vi "operationFunction.vi"(1 "y":dbl, 2 "Operation":string(combo), 3 "x":dbl) -> (0 "Answer":dbl)   [LabVIEW 2018]
panel:
  out "Units":string
  in  "stop":bool
  out "Error Message":string
  in  "Radians/Degrees":bool
  out "Operation Taken":string
  # "Tom's Calculator"
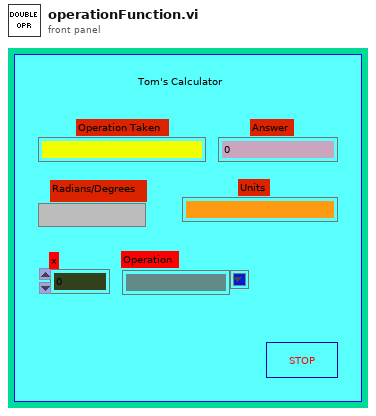
[diagram p1: front panel]
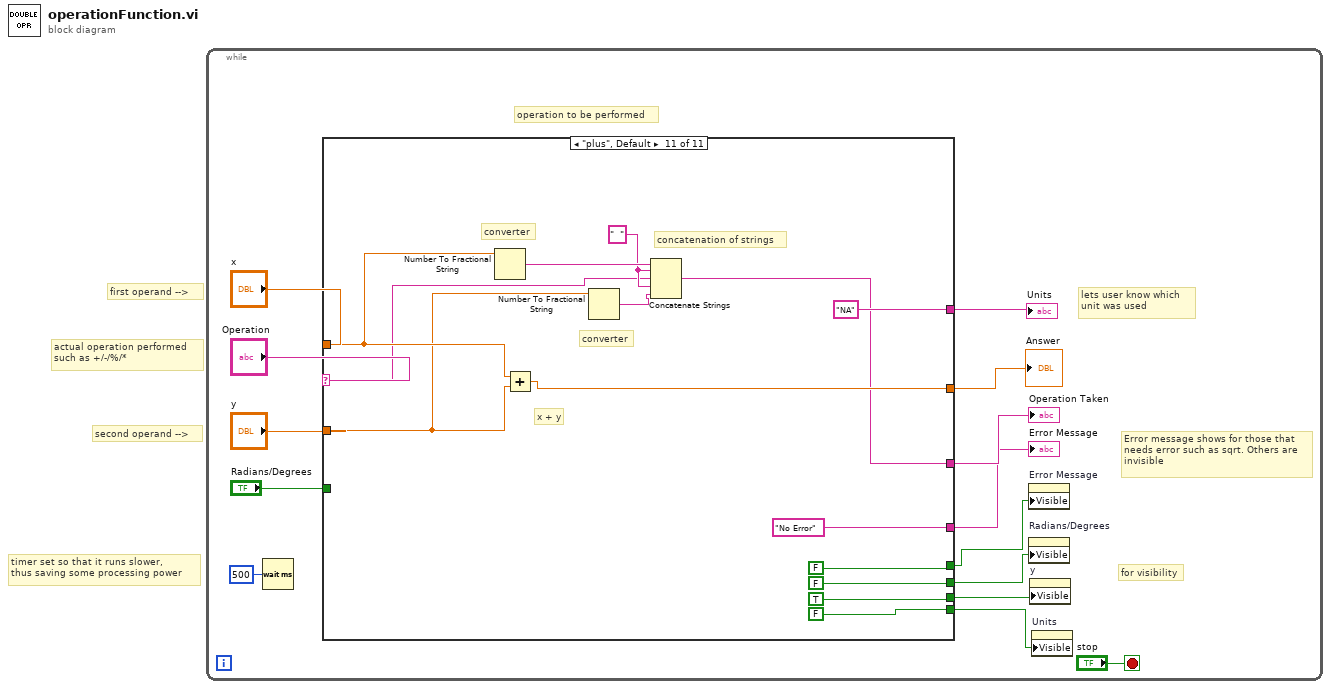
[diagram p0: block diagram]
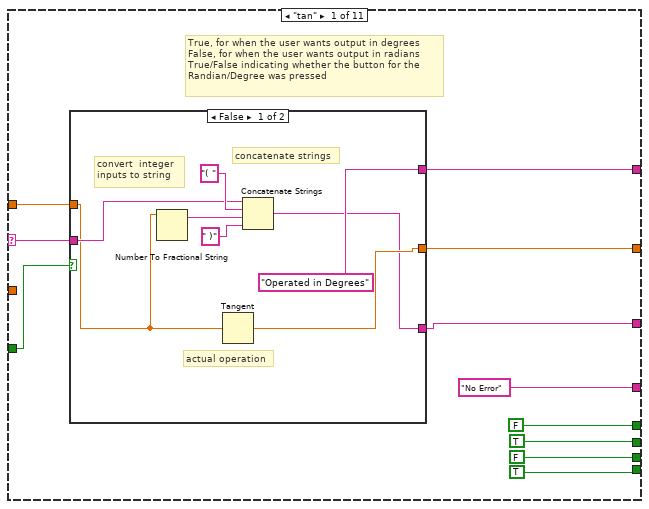
[diagram p2: hidden frame]
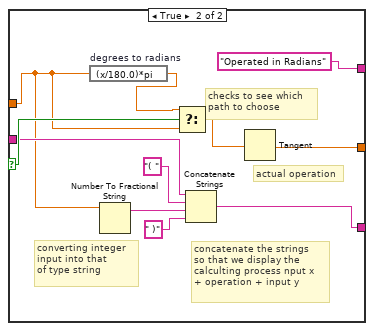
[diagram p3: hidden frame]
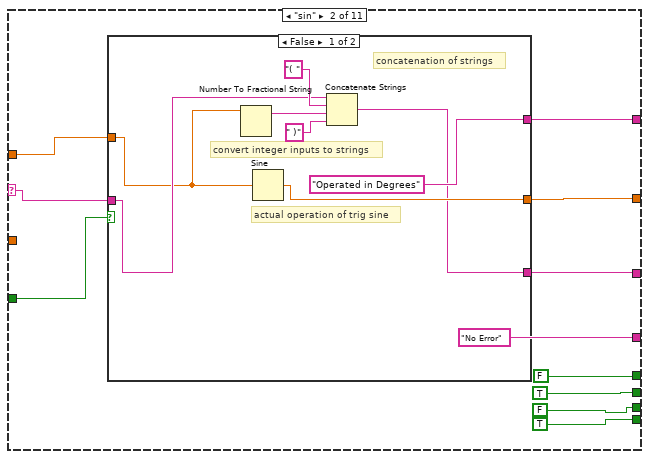
[diagram p4: hidden frame]
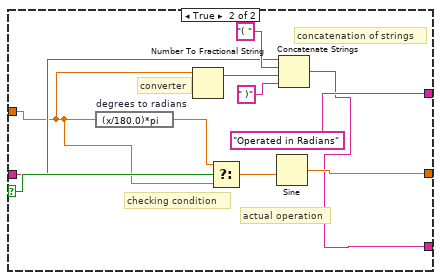
[diagram p5: hidden frame]
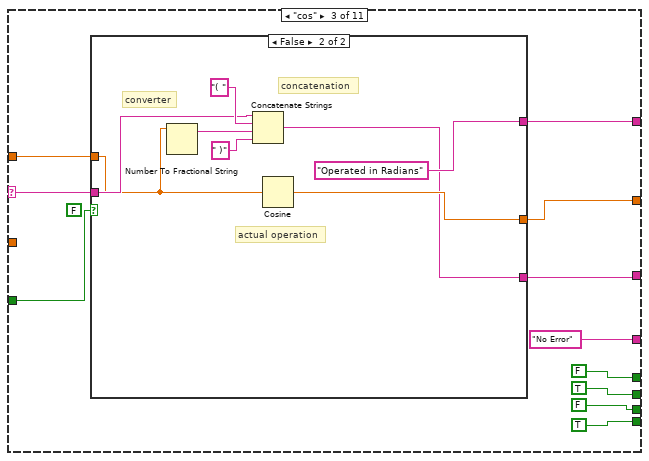
[diagram p6: hidden frame]
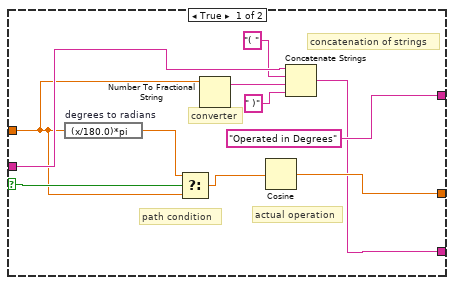
[diagram p7: hidden frame]
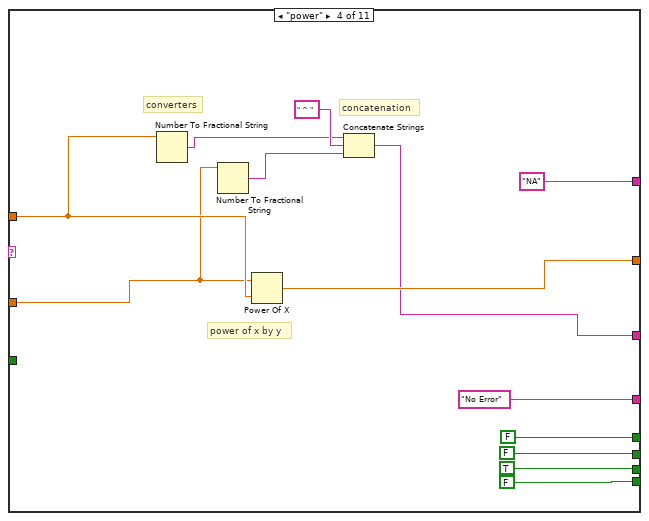
[diagram p8: hidden frame]
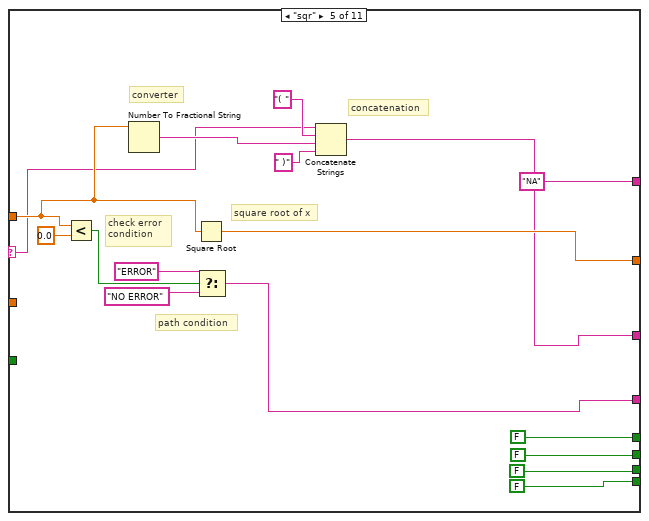
[diagram p9: hidden frame]
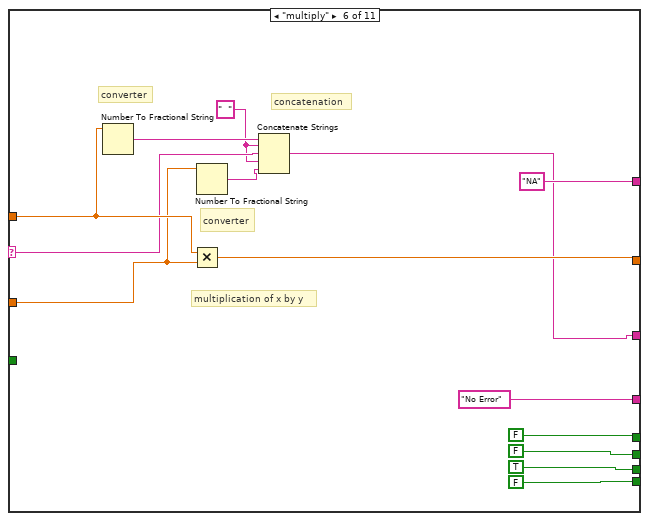
[diagram p10: hidden frame]
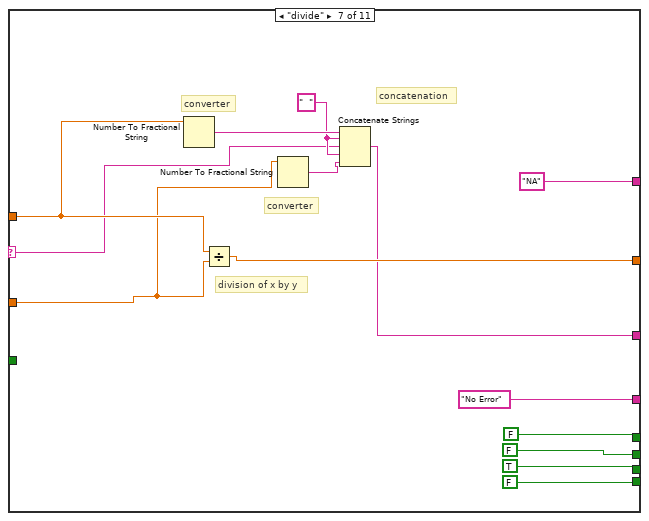
[diagram p11: hidden frame]
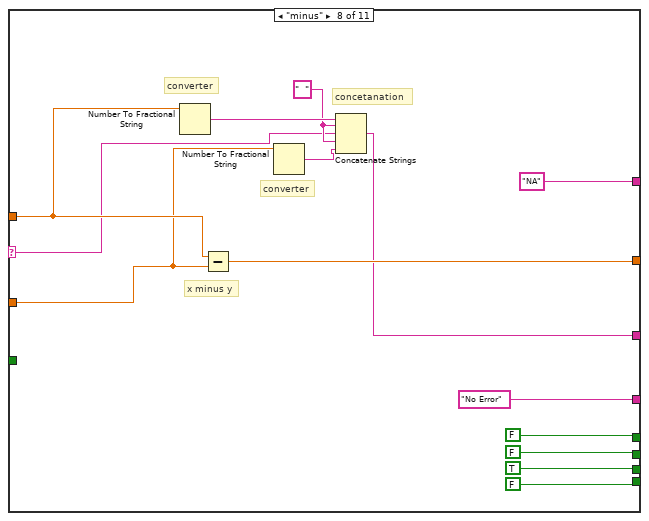
[diagram p12: hidden frame]
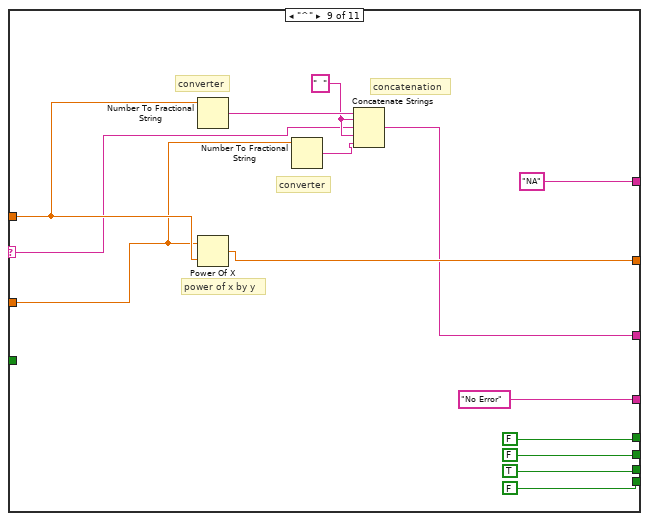
[diagram p13: hidden frame]
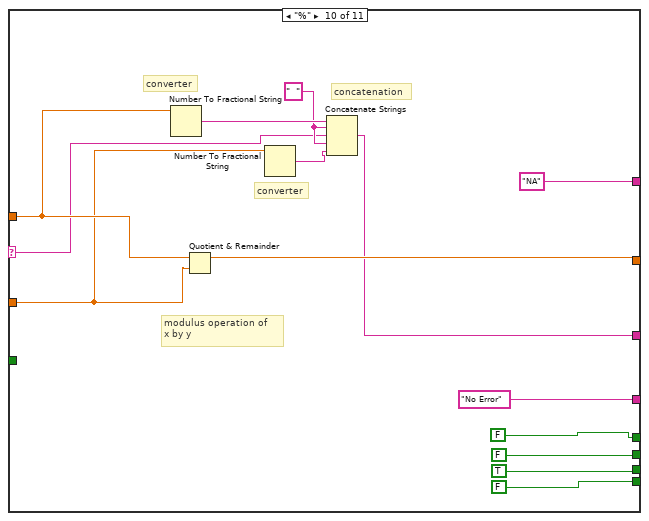
[diagram p14: hidden frame]
diagram:
  # "timer set so that it runs slower,\nthus saving some processing power"
  # "actual operation performed \nsuch as +/-/%/*"
  # "second operand -->"
  # "first operand -->"
  n1 = while {
    stop <- "stop" stop-if-true
    # "for visibility"
    # "Error message shows for those that \nneeds error such as sqrt. Others are \ninvisible"
    # "lets user know which \nunit was used"
    # "operation to be performed"
    n2 = Wait (ms)(milliseconds to wait=u32 500) -> ()  [unwired: 1 out]
    n3 = case shown="\"plus\", Default" "Operation" {
      selector: "Operation" -> [w16 w52 w76 _ w118 w137 w151 w165 w178 w193 w205]
      tunnel: "x" -> [w25 w54 w85 w109 w122 w141 w152 w166 w180 w194 w208]
      tunnel: "y" -> [_ _ _ w107 _ w139 w150 w164 w179 w192 w207]
      tunnel: [w24 w55 w84 w117 w132 w148 w162 w176 w190 w204 w218] -> w10
      tunnel: [w15 w50 w75 w105 w119 w138 w149 w163 w177 w191 w206] -> w11
      tunnel: ["No Error" "No Error" "No Error" "No Error" w129 "No Error" "No Error" "No Error" "No Error" "No Error" "No Error"] -> w9
      tunnel: "Radians/Degrees" -> [w22 w51 w82 _ _ _ _ _ _ _ _]
      tunnel: [w21 w49 w81 "NA" "NA" "NA" "NA" "NA" "NA" "NA" "NA"] -> w5
      tunnel: [FALSE FALSE FALSE TRUE FALSE TRUE TRUE TRUE TRUE TRUE TRUE] -> w4
      tunnel: [TRUE TRUE TRUE FALSE FALSE FALSE FALSE FALSE FALSE FALSE FALSE] -> w3
      tunnel: [TRUE TRUE TRUE FALSE FALSE FALSE FALSE FALSE FALSE FALSE FALSE] -> w2
      tunnel: [FALSE FALSE FALSE FALSE FALSE FALSE FALSE FALSE FALSE FALSE FALSE] -> w1
      frame "tan" {
        # "True, for when the user wants output in degrees\nFalse, for when the user wants output in radians\nTrue/False indicating whether the button for the\nRandian/Degree was pressed"
        n4 = case shown="False" w22 {
          selector: w22 -> [_ w43]
          tunnel: w25 -> [w26 w34]
          tunnel: [w33 w44] -> w24
          tunnel: ["Operated in Degrees" "Operated in Radians"] -> w21
          tunnel: w16 -> [w28 w36]
          tunnel: [w27 w35] -> w15
          frame False {
            # "actual operation"
            # "convert  integer \ninputs to string"
            # "concatenate strings"
            n5 = Number To Fractional String(number=w26) -> (F-format string=w31:string)  [unwired: 3 in]
            n6 = Tangent(1:w26) -> (0:w33:dbl)
            n7 = Concatenate Strings(w28, "( " ("string"), w31, " )" ("string")) -> (w27:string)
          }
          frame True {
            # "converting integer \ninput into that \nof type string"
            # "actual operation"
            # "checks to see which \npath to choose"
            # "concatenate the strings\nso that we display the \ncalculting process nput x \n+ operation + input y"
            n8 = expression code="(x/180.0)*pi" "degrees to radians"(w34) -> (w42:dbl)
            n9 = Number To Fractional String(number=w34) -> (F-format string=w39:string)  [unwired: 3 in]
            n10 = Select(t=w42, s=w43, f=w34) -> (s? t:f=w41:dbl)
            n11 = Concatenate Strings(w36, "( " ("string"), w39, " )" ("string")) -> (w35:string)
            n12 = Tangent(1:w41) -> (0:w44:dbl)
          }
        }
      }
      frame "sin" {
        n13 = case shown="False" w51 {
          selector: w51 -> [_ w71]
          tunnel: [w63 w74] -> w55
          tunnel: w54 -> [w56 w65]
          tunnel: w52 -> [w58 w66]
          tunnel: [w57 w64] -> w50
          tunnel: ["Operated in Degrees" "Operated in Radians"] -> w49
          frame False {
            # "actual operation of trig sine"
            # "convert integer inputs to strings"
            # "concatenation of strings"
            n14 = Number To Fractional String(number=w56) -> (F-format string=w61:string)  [unwired: 3 in]
            n15 = Sine(x=w56) -> (sin(x)=w63:dbl)
            n16 = Concatenate Strings(w58, "( " ("string"), w61, " )" ("string")) -> (w57:string)
          }
          frame True {
            # "concatenation of strings"
            # "converter"
            # "checking condition"
            # "actual operation"
            n17 = expression code="(x/180.0)*pi" "degrees to radians"(w65) -> (w73:dbl)
            n18 = Number To Fractional String(number=w65) -> (F-format string=w69:string)  [unwired: 3 in]
            n19 = Select(t=w73, s=w71, f=w65) -> (s? t:f=w72:dbl)
            n20 = Sine(x=w72) -> (sin(x)=w74:dbl)
            n21 = Concatenate Strings(w66, "( " ("string"), w69, " )" ("string")) -> (w64:string)
          }
        }
      }
      frame "cos" {
        (unwired) FALSE
        n22 = case shown="False" w82 {
          selector: w82 -> [w96 _]
          tunnel: w85 -> [w86 w98]
          tunnel: [w94 w104] -> w84
          tunnel: ["Operated in Degrees" "Operated in Radians"] -> w81
          tunnel: [w87 w97] -> w75
          tunnel: w76 -> [w90 w99]
          frame True {
            # "concatenation of strings"
            # "converter"
            # "actual operation"
            # "path condition"
            n23 = expression code="(x/180.0)*pi" "degrees to radians"(w86) -> (w95:dbl)
            n24 = Select(t=w95, s=w96, f=w86) -> (s? t:f=w88:dbl)
            n25 = Number To Fractional String(number=w86) -> (F-format string=w92:string)  [unwired: 3 in]
            n26 = Cosine(x=w88) -> (cos(x)=w94:dbl)
            n27 = Concatenate Strings(w90, "( " ("string"), w92, " )" ("string")) -> (w87:string)
          }
          frame False {
            # "concatenation"
            # "converter"
            # "actual operation"
            n28 = Number To Fractional String(number=w98) -> (F-format string=w102:string)  [unwired: 3 in]
            n29 = Concatenate Strings(w99, "( " ("string"), w102, " )" ("string")) -> (w97:string)
            n30 = Cosine(x=w98) -> (cos(x)=w104:dbl)
          }
        }
      }
      frame "power" {
        # "concatenation"
        # "converters"
        # "power of x by y"
        n31 = Number To Fractional String(number=w109) -> (F-format string=w108:string)  [unwired: 3 in]
        n32 = Number To Fractional String(number=w107) -> (F-format string=w106:string)  [unwired: 3 in]
        n33 = Power Of X(1:w109, 2:w107) -> (0:w117:dbl)
        n34 = Concatenate Strings(w108, " ^ " ("string"), w106) -> (w105:string)
      }
      frame "sqr" {
        # "check error \ncondition"
        # "square root of x"
        # "path condition"
        # "converter"
        # "concatenation"
        n35 = Less?(x=w122, y=0.0) -> (x < y?=w133:bool)
        n36 = Number To Fractional String(number=w122) -> (F-format string=w121:string)  [unwired: 3 in]
        n37 = Square Root(x=w122) -> (sqrt(x)=w132:dbl)
        n38 = Select(t="ERROR", s=w133, f="NO ERROR") -> (s? t:f=w129:string)
        n39 = Concatenate Strings(w118, "( " ("string"), w121, " )" ("string")) -> (w119:string)
      }
      frame "multiply" {
        w136 = "  " ("string")
        # "multiplication of x by y"
        # "converter"
        # "converter"
        # "concatenation"
        n40 = Number To Fractional String(number=w141) -> (F-format string=w140:string)  [unwired: 3 in]
        n41 = Multiply(x=w141, y=w139) -> (x*y=w148:dbl)
        n42 = Number To Fractional String(number=w139) -> (F-format string=w135:string)  [unwired: 3 in]
        n43 = Concatenate Strings(w140, w136, w137, w136, w135) -> (w138:string)
      }
      frame "divide" {
        w154 = "  " ("string")
        # "division of x by y"
        # "converter"
        # "converter"
        # "concatenation"
        n44 = Number To Fractional String(number=w152) -> (F-format string=w155:string)  [unwired: 3 in]
        n45 = Divide(x=w152, y=w150) -> (x/y=w162:dbl)
        n46 = Number To Fractional String(number=w150) -> (F-format string=w153:string)  [unwired: 3 in]
        n47 = Concatenate Strings(w155, w154, w151, w154, w153) -> (w149:string)
      }
      frame "minus" {
        w168 = "  " ("string")
        # "x minus y"
        # "concetanation"
        # "converter"
        # "converter"
        n48 = Number To Fractional String(number=w166) -> (F-format string=w169:string)  [unwired: 3 in]
        n49 = Subtract(x=w166, y=w164) -> (x-y=w176:dbl)
        n50 = Number To Fractional String(number=w164) -> (F-format string=w167:string)  [unwired: 3 in]
        n51 = Concatenate Strings(w169, w168, w165, w168, w167) -> (w163:string)
      }
      frame "^" {
        w182 = "  " ("string")
        # "concatenation"
        # "converter"
        # "converter"
        # "power of x by y"
        n52 = Number To Fractional String(number=w180) -> (F-format string=w183:string)  [unwired: 3 in]
        n53 = Power Of X(1:w180, 2:w179) -> (0:w190:dbl)
        n54 = Number To Fractional String(number=w179) -> (F-format string=w181:string)  [unwired: 3 in]
        n55 = Concatenate Strings(w183, w182, w178, w182, w181) -> (w177:string)
      }
      frame "%" {
        w196 = "  " ("string")
        # "modulus operation of \nx by y"
        # "converter"
        # "converter"
        # "concatenation"
        n56 = Number To Fractional String(number=w194) -> (F-format string=w197:string)  [unwired: 3 in]
        n57 = Quotient & Remainder(x=w194, y=w192) -> (x-y*floor(x/y)=w204:dbl)  [unwired: 1 out]
        n58 = Number To Fractional String(number=w192) -> (F-format string=w195:string)  [unwired: 3 in]
        n59 = Concatenate Strings(w197, w196, w193, w196, w195) -> (w191:string)
      }
      frame "plus", Default {
        w210 = "  " ("string")
        # "concatenation of strings"
        # "converter"
        # "converter"
        # "x + y"
        n60 = Number To Fractional String(number=w208) -> (F-format string=w211:string)  [unwired: 3 in]
        n61 = Add(x=w208, y=w207) -> (x+y=w218:dbl)
        n62 = Number To Fractional String(number=w207) -> (F-format string=w209:string)  [unwired: 3 in]
        n63 = Concatenate Strings(w211, w210, w205, w210, w209) -> (w206:string)
      }
    }
    "Answer" <- w10
    "Operation Taken" <- w11
    "Error Message" <- w9
    "Units" <- w5
    n64 = property on="Error Message" class="Str"("Visible"=w1) -> ()  [unwired: 2 in, 2 out]
    n65 = property on="Radians/Degrees" class="Bool (strict)"("Visible"=w2) -> ()  [unwired: 2 in, 2 out]
    n66 = property on="y" class="DigNum (strict)"("Visible"=w4) -> ()  [unwired: 2 in, 2 out]
    n67 = property on="Units" class="Str"("Visible"=w3) -> ()  [unwired: 2 in, 2 out]
  }
